vi "Synthesize Pulse.vi"(0 "Pulse Train in":refnum<class "Pulse Train.lvclass">, 9 "Fs (Hz)":dbl, 11 "error in (no error)":errorcluster) -> (4 "Pulse Train out":refnum<class "Pulse Train.lvclass">, 8 "Pulse":dbl[](array[numeric]), 15 "error out":errorcluster)   [LabVIEW 2015, in "Pulse Train.lvclass"]
uses:
  Pulse Train.lvclass
  Pulse Train.lvclass/Pulse Train.ctl
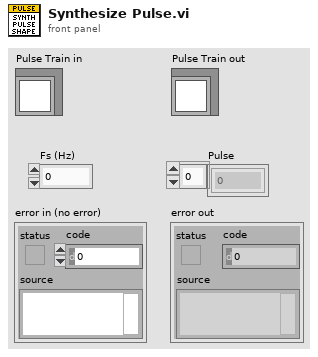
[diagram p1: front panel]
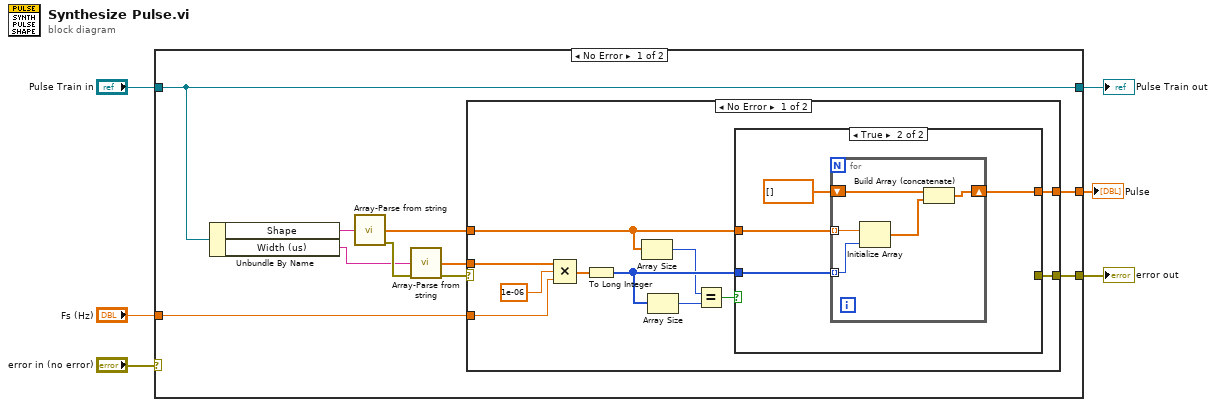
[diagram p0: block diagram]
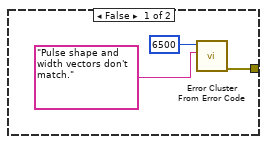
[diagram p2: hidden frame]
diagram:
  n1 = case shown="No Error" "error in (no error)" {
    selector: "error in (no error)" -> [_ w42]
    tunnel: [w7 w42] -> w5
    tunnel: [w16 w41] -> w3
    tunnel: "Pulse Train in" -> [w16 w41]
    tunnel: "Fs (Hz)" -> [w11 _]
    tunnel: [w10 _] -> w1
    frame No Error {
      n2 = Unbundle By Name(w16) -> ("Shape"=w15:string, "Width (us)"=w13:string)
      n3 = call "Array-Parse from string.vi"("String"=w15) -> ("Array"=w9:dbl[], "error out"=w14:errorcluster)  [unwired: 13 in]
      n4 = call "Array-Parse from string.vi"("String"=w13, "error in (no error)"=w14) -> ("Array"=w12:dbl[], "error out"=w8:errorcluster)  [unwired: 12 in]
      n5 = case shown="No Error" w8 {
        selector: w8 -> [_ w40]
        tunnel: w12 -> [w27 _]
        tunnel: w11 -> [w26 _]
        tunnel: [w23 _] -> w10
        tunnel: w9 -> [w22 _]
        tunnel: [w17 w40] -> w7
        frame No Error {
          n6 = Compound Arithmetic op=MULTIPLY(w27, 1e-06 ("value"), w26) -> (w24:dbl[])
          n7 = To Long Integer(number=w24) -> (32bit integer=w21:i32[])
          n8 = Array Size(array=w22) -> (size(s)=w19:i32)
          n9 = Array Size(array=w21) -> (size(s)=w20:i32)
          n10 = Equal?(x=w19, y=w20) -> (x = y?=w18:bool)
          n11 = case shown="True" w18 {
            tunnel: [_ w34] -> w23
            tunnel: w22 -> [_ w32]
            tunnel: w21 -> [_ w31]
            tunnel: [w30 _] -> w17
            frame False {
              n12 = call <vilib>:"Error Cluster From Error Code.vi"("error message (\"\")"="Pulse shape and width vectors don't match." ("error message (\"\")"), "error code (0)"=6500) -> ("error out"=w30:errorcluster)  [unwired: 7 in]
            }
            frame True {
              n13 = for {
                shift-right: [w35] -> w34
                shift-left: dbl[] [] -> [w37]
                tunnel: w31 -> [w39] mode=indexing
                tunnel: w32 -> [w38] mode=indexing
                n14 = Initialize Array(w38, w39) -> (w36:dbl[])
                n15 = Build Array (concatenate)(w37, w36) -> (w35:dbl[])
              }
            }
          }
        }
        frame Error {
        }
      }
    }
    frame Error {
    }
  }
  "error out" <- w5
  "Pulse Train out" <- w3
  "Pulse" <- w1
